vi "IL-Sensor Setting.vi"() -> (1 "IL Sensor":T1, 3 "Search Key":string)   [LabVIEW 2015]
uses:
  Galobal variable_TI.vi
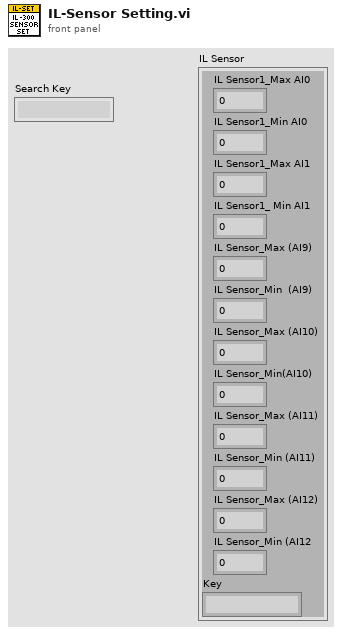
[diagram p1: front panel]
types:
  T1 = cluster{"IL Sensor1_Max AI0":dbl, "IL Sensor1_Min AI0":dbl, "IL Sensor1_Max AI1":dbl, "IL Sensor1_ Min AI1":dbl, "IL Sensor_Max (AI9)":dbl, "IL Sensor_Min  (AI9)":dbl, "IL Sensor_Max (AI10)":dbl, "IL Sensor_Min(AI10)":dbl, "IL Sensor_Max (AI11)":dbl, "IL Sensor_Min (AI11)":dbl, "IL Sensor_Max (AI12)":dbl, "IL Sensor_Min (AI12":dbl, "Key":string}
  T2 = cluster{"IL Sensor1_Max AI0":dbl, "IL Sensor1_Min AI0":dbl, "IL Sensor1_Max AI1":dbl, "IL Sensor1_ Min AI1":dbl, "IL Sensor_Max (AI9)":dbl, "IL Sensor_Min  (AI9)":dbl, "IL Sensor_Max (AI10)":dbl, "IL Sensor_Min(AI10)":dbl, "IL Sensor_Max (AI11)":dbl, "IL Sensor_Min (AI11)":dbl, "IL Sensor_Max (AI12)":dbl, "IL Sensor_Min (AI12":dbl}
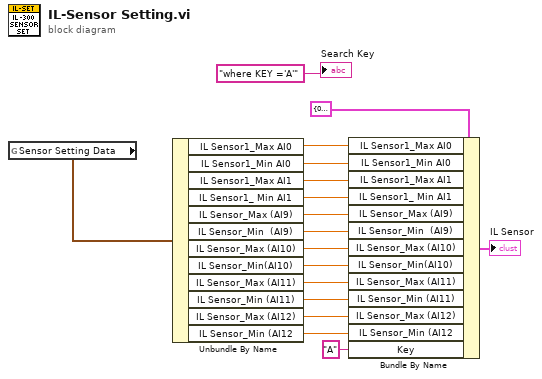
[diagram p0: block diagram]
diagram:
  n1 = global read "Galobal variable_TI.vi" "Sensor Setting Data"() -> (w16:T2)
  n2 = Unbundle By Name(w16) -> ("IL Sensor1_Max AI0"=w17:dbl, "IL Sensor1_Min AI0"=w13:dbl, "IL Sensor1_Max AI1"=w12:dbl, "IL Sensor1_ Min AI1"=w11:dbl, "IL Sensor_Max (AI9)"=w10:dbl, "IL Sensor_Min  (AI9)"=w9:dbl, "IL Sensor_Max (AI10)"=w8:dbl, "IL Sensor_Min(AI10)"=w7:dbl, "IL Sensor_Max (AI11)"=w6:dbl, "IL Sensor_Min (AI11)"=w5:dbl, "IL Sensor_Max (AI12)"=w4:dbl, "IL Sensor_Min (AI12"=w3:dbl)
  n3 = Bundle By Name(cluster=T1 {"IL Sensor1_Max AI0"=0.0, "IL Sensor1_Min AI0"=0.0, "IL Sensor1_Max AI1"=0.0, "IL Sensor1_ Min AI1"=0.0, "IL Sensor_Max (AI9)"=0.0, "IL Sensor_Min  (AI9)"=0.0, "IL Sensor_Max (AI10)"=0.0, "IL Sensor_Min(AI10)"=0.0, "IL Sensor_Max (AI11)"=0.0, "IL Sensor_Min (AI11)"=0.0, "IL Sensor_Max (AI12)"=0.0, "IL Sensor_Min (AI12"=0.0, "Key"=""} ("Sensor Setting Data 2"), "IL Sensor1_Max AI0"=w17, "IL Sensor1_Min AI0"=w13, "IL Sensor1_Max AI1"=w12, "IL Sensor1_ Min AI1"=w11, "IL Sensor_Max (AI9)"=w10, "IL Sensor_Min  (AI9)"=w9, "IL Sensor_Max (AI10)"=w8, "IL Sensor_Min(AI10)"=w7, "IL Sensor_Max (AI11)"=w6, "IL Sensor_Min (AI11)"=w5, "IL Sensor_Max (AI12)"=w4, "IL Sensor_Min (AI12"=w3, "Key"="A") -> (→"IL Sensor":T1)
  "Search Key" <- "where KEY ='A'"
